vi "ProcessCompletionWaiter (SubVI).vi"(11 "VISA Refnum in":refnum<visa-resource-name>) -> ()   [LabVIEW 2020]
panel:
  out "Process Status":bool
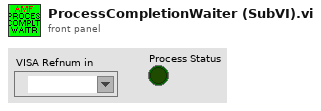
[diagram p1: front panel]
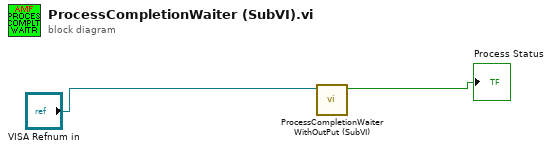
[diagram p0: block diagram]
diagram:
  n1 = call "ProcessCompletionWaiterWithOutPut (SubVI).vi"("VISA Refnum in"="VISA Refnum in") -> ("Boolean"=→"Process Status":bool)  [unwired: 10 in]
